vi "SetParam.vi"(8 "error in (no error)":errorcluster caption="entrée d'erreur (pas d'erreur)", 10 "cohen_kappa_score":T1={"labels"=[], "weights"="None", "sample_weight"=[]}, 11 "Cohen_Kappa_Score.lvclass":refnum<class "Cohen_Kappa_Score.lvclass">) -> (0 "error out":errorcluster caption="sortie d'erreur", 3 "Cohen_Kappa_Score.lvclass":refnum<class "Cohen_Kappa_Score.lvclass">)   [LabVIEW 2020, in "Cohen_Kappa_Score.lvclass"]
doc: "Set Parameters"
uses:
  Cohen_Kappa_Score.lvclass
  Cohen_Kappa_Score.lvclass/Cohen_Kappa_Score.ctl
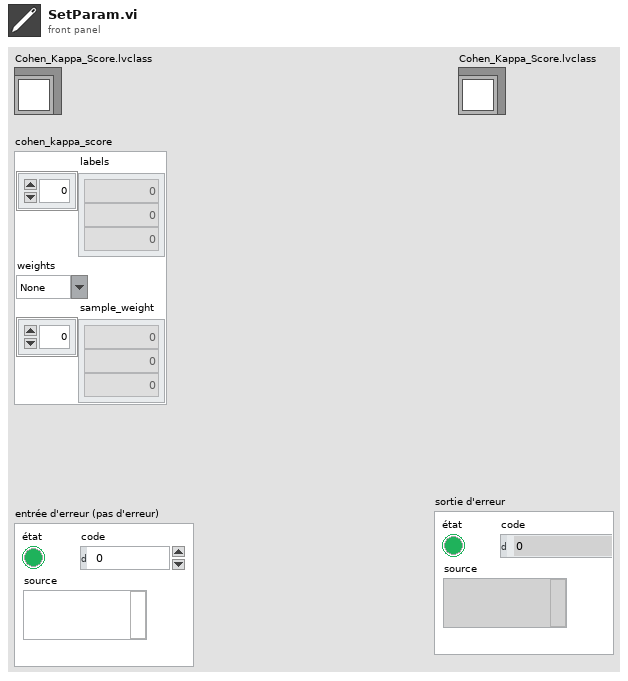
[diagram p1: front panel]
types:
  T1 = cluster{"labels":i32[], "weights":string, "sample_weight":dbl[]}
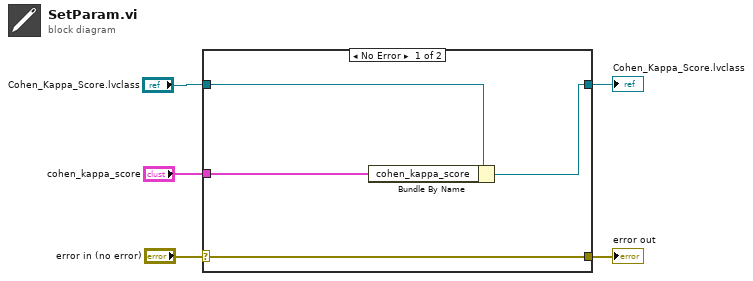
[diagram p0: block diagram]
diagram:
  n1 = case shown="No Error" "error in (no error)" {
    selector: "error in (no error)" -> [w9 w10]
    tunnel: [w9 w10] -> w4
    tunnel: [w7 w11] -> w2
    tunnel: "Cohen_Kappa_Score.lvclass" -> [w8 w11]
    tunnel: "cohen_kappa_score" -> [w6 _]
    frame No Error {
      n2 = Bundle By Name(cluster=w8, "cohen_kappa_score"=w6) -> (w7:refnum<class "Cohen_Kappa_Score.lvclass">)
    }
    frame Error {
    }
  }
  "error out" <- w4
  "Cohen_Kappa_Score.lvclass" <- w2
